vi "Test_LogValueEvent_LogMultipleDBLandTime_MatchFormattoString.vi"(8 "error in (no error)":errorcluster, 11 "TestCase in":refnum<class "TestLogValue.lvclass">) -> (0 "error out":errorcluster, 3 "TestCase out":refnum<class "TestLogValue.lvclass">)   [LabVIEW 2019, in "TestLogValue.lvclass"]
uses:
  TestLogValue.lvclass
  Source/Composed Log/Types/Log Level.ctl
  Source/Composed Log/LoggerReference/LoggerReference.lvclass/LoggerReference.ctl
  Source/LVQueue Sink/LVQueue Sink.lvclass/LVQueue Sink.ctl
  272d61b2-f49c-486c-9daf-337ffb054b40.vi
  154dbc8a-62f5-4aa1-ad82-2a3c469f95b7.vi
  Source/Composed Log/LoggerReference/Return Aggregate Queues.vi
  Source/Composed Log/LoggerReference/Add Aggregate Log.vi
  272d61b2-f49c-486c-9daf-337ffb054b40.vi/935b51ff-062d-440a-bc79-c49c54825b54.vi
  154dbc8a-62f5-4aa1-ad82-2a3c469f95b7.vi/02efea92-9ff9-467e-b72d-ce5ac48a1fd5.vi
  Source/Composed Log/LoggerReference/Get Formatter.vi
  Source/Composed Log/LoggerReference/Get Valid Event Time.vi
  Source/Composed Log/LoggerReference/Log Event.vi
  Source/Composed Log/LoggerReference/Send Add Sink.vi
  Source/Composed Log/LoggerReference/Log.vi
  Source/Composed Log/LoggerReference/Remove Stale Logs.vi
  Source/LVQueue Sink/LVQueue Sink.lvclass
  C:/CS/Log/Source/Composed Log/Log Sink/Log Sink.lvclass
  Source/Composed Log/Application Logger/Launch Worker Loop.vi
  Source/Composed Log/LoggerReference/Initialize Logger Instance.vi
  Source/Composed Log/LoggerReference/Format Variant.vi
  Source/Composed Log/LoggerReference/LoggerReference.lvclass
  Source/Composed Log/IErrorFormat/IErrorFormat.lvclass
  Source/Composed Log/Log Sink/Log Sink.lvclass
  <vilib>/addons/_JKI Toolkits/VI Tester/TestCase.llb/TestCase.lvclass
  Source/Composed Log/Composed Log.lvlib
  C:/Program Files (x86)/National Instruments/LabVIEW 2019/vi.lib/addons/_JKI Toolkits/VI Tester/TestCase.llb/TestCase.lvclass
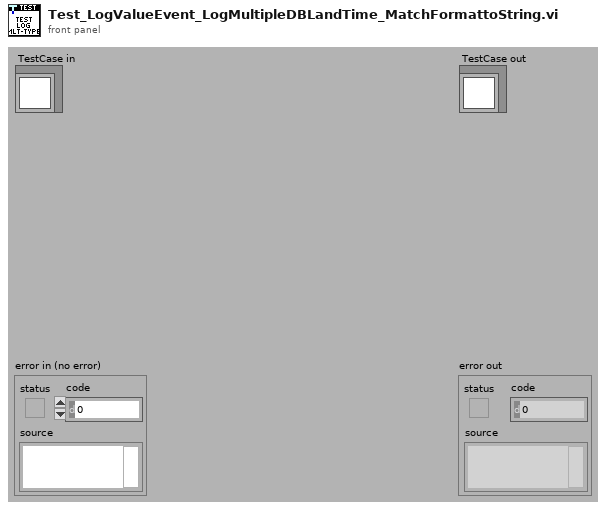
[diagram p1: front panel]
types:
  T1 = typedef "Composed Log.lvlib/Log Level.ctl" = enum16{"Debug", "Info", "Warning", "Error", "Critical"}
  T2 = typedef "Composed Log.lvlib/Log Packet.ctl" = cluster{"Data To Log":string, "Source":string, "Event Level":T1, "Event Time":timestamp}
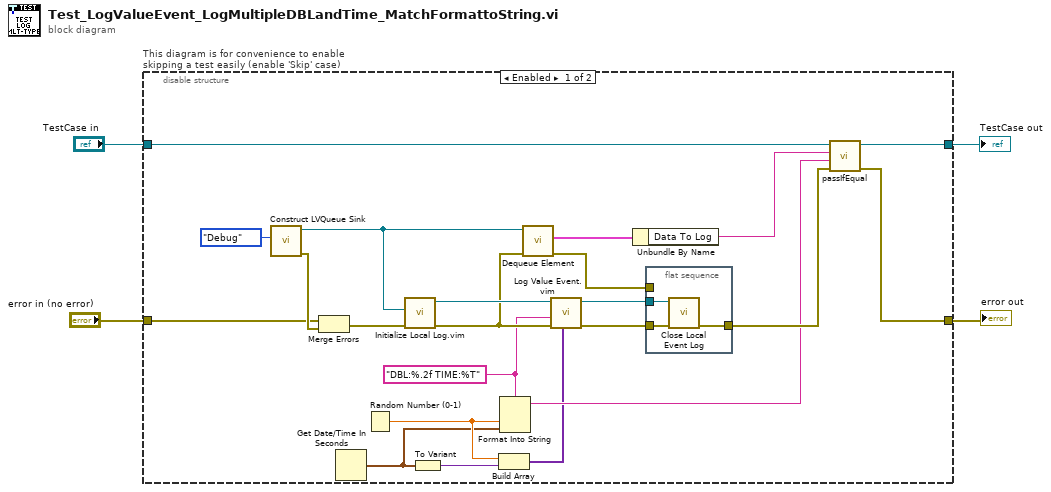
[diagram p0: block diagram]
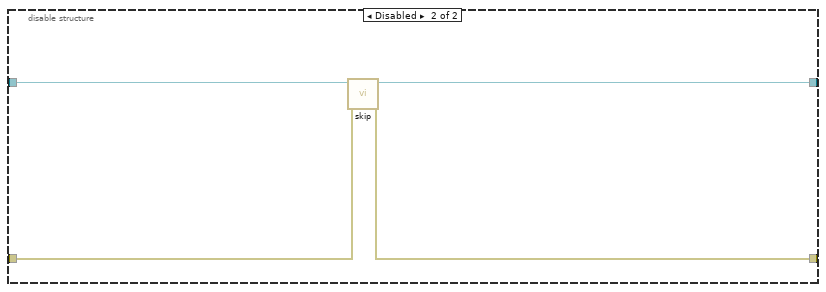
[diagram p2: hidden frame]
diagram:
  n1 = disable-structure "This diagram is for convenience to enable skipping a test easily (enable 'Skip' case)" shown="Enabled" {
    disable-tunnel: "TestCase in" -> [w20 w33]
    disable-tunnel: [w19 w31] -> w1
    disable-tunnel: [w17 w32] -> w3
    disable-tunnel: "error in (no error)" -> [w18 w30]
    frame Enabled {
      w12 = "DBL:%.2f TIME:%T" ("Data To Log")
      n2 = call "Construct LVQueue Sink.vi"("LogLevel"=Log_Level."Debug") -> ("error out"=w23:errorcluster, "LVQueue Sink out"=w21:refnum<class "LVQueue Sink.lvclass">)  [unwired: 9 in]
      n3 = Merge Errors(w18, w23) -> (w22:errorcluster)
      n4 = Get Date/Time In Seconds() -> (seconds since 1Jan1904=w5:timestamp)
      n5 = Random Number (0-1)() -> (number: 0 to 1=w8:dbl)
      n6 = call "Initialize Local Log.vim"("error in (no error)"=w22, "Startup Sink(s)"=w21) -> ("error out"=w15:errorcluster, "Log Instance Reference"=w16:refnum<class "LoggerReference.lvclass">)  [unwired: 7 in, 1 out]
      n7 = To Variant(anything=w5) -> (Variant=w6:variant)
      n8 = Build Array(w8, w6) -> (w7:variant[])
      n9 = Format Into String(format string=w12, w8, w5) -> (resulting string=w10:string)  [unwired: 2 in, 1 out]
      n10 = call "Dequeue Element.vi"("error in (no error)"=w15, "LVQueue Sink in"=w21) -> ("error out"=w26:errorcluster, "Log Packet"=w24:T2)  [unwired: 6 in, 2 out]
      n11 = call "Log Value Event.vim"("Value(s)"=w7, "error in (no error)"=w15, "Log Message Format String"=w12, "LoggerReference in"=w16) -> ("error out"=w14:errorcluster, "LoggerReference out"=w13:refnum<class "LoggerReference.lvclass">)  [unwired: 6 in]
      n12 = Unbundle By Name(w24) -> ("Data To Log"=w11:string)
      n13 = flat-sequence {
        tunnel: [w28] -> w25
        tunnel: w14 -> [w29]
        tunnel: w26 -> [_]
        tunnel: w13 -> [w27]
        frame #0 {
          n14 = call "Close Local Event Log.vi"("error in (no error)"=w29, "Log Instance"=w27) -> ("error out"=w28:errorcluster)  [unwired: 9 in]
        }
      }
      n15 = call-dynamic "passIfEqual.vi"("error in (no error)"=w25, "y"=w10, "x"=w11, "TestCase in"=w20) -> ("error out"=w17:errorcluster, "TestCase out"=w19:refnum<class "TestLogValue.lvclass">)  [unwired: 6 in]
    }
    frame Disabled {
      # "skip test result while test is under development"
      n16 = call <vilib>:"skip.vi"("error in (no error)"=w30, "TestCase in"=w33) -> ("error out"=w32:errorcluster, "TestCase out"=w31:refnum<class "TestLogValue.lvclass">)  [unwired: 8 in]
    }
  }
  "error out" <- w3
  "TestCase out" <- w1
